vi "Fetch Multi Eval Meas List Segment Modulation Results.vi"(6 "Segment (1)":T2=1, 8 "error in (no error)":errorcluster, 9 "Result Type (Current)":i32(ring) items=["Current"=0, "Average"=1, "Standard Deviation"=3], 10 "Instance (1)":T3=1, 11 "VISA resource name":refnum<visa-resource-name>) -> (0 "error out":errorcluster, 1 "Results":dbl[](array[numeric]) format="%^.3e", 2 "Reliability":T1, 3 "VISA resource name out":refnum<visa-resource-name>, 4 "Expired Statistics":i32, 5 "Out Of Tolerance":i32)   [LabVIEW 2020, in "Rohde&Schwarz CMWXP NR FR1 Measurement.lvlib"]
doc: "Returns modulation single value results for segment <no> in list mode.\n\nAttributes:\nRSCMWXPNRFR1M_ATTR_FETCH_MULTI_EVAL_MEAS_LIST_SEGMENT_MODULATION_CURRENT_RESULTS\nRSCMWXPNRFR1M_ATTR_FETCH_MULTI_EVAL_MEAS_LIST_SEGMENT_MODULATION_AVERAGE_RESULTS\nRSCMWXPNRFR1M_ATTR_FETCH_MULTI_EVAL_MEAS_LIST_SEGMENT_MODULATION_STANDARD_DEVIATION_RESULTS\n\nRemote-control commands:\nFETCh:NRSub:MEAS<i>:MEValuation:LIST:SEGMent<no>:MODulation:CURRent?\nFETCh:NRSub:MEAS<i>:MEValuation:LIST:SEGMent<no>:MODulation:AVERage?\nFETCh:NRSub:MEAS<i>:MEValuation:LIST:SEGMent<no>:MODulation:SDEViation?"
uses:
  <instrlib>/Rohde&Schwarz CMWXP NR FR1 Measurement/Rohde&Schwarz CMWXP NR FR1 Measurement.lvlib
  <instrlib>/Rohde&Schwarz CMWXP NR FR1 Measurement/Private/_Instance.ctl
  <instrlib>/Rohde&Schwarz CMWXP NR FR1 Measurement/Private/_Segment.ctl
  <instrlib>/Rohde&Schwarz CMWXP NR FR1 Measurement/Private/_SegReliability.ctl
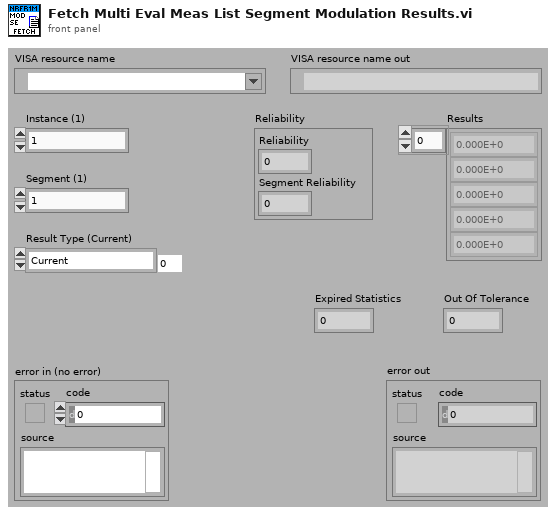
[diagram p1: front panel]
types:
  T1 = typedef "Rohde&Schwarz CMWXP NR FR1 Measurement.lvlib/_SegReliability.ctl" = cluster{"Reliability":i32, "Segment Reliability":i32}
  T2 = typedef "Rohde&Schwarz CMWXP NR FR1 Measurement.lvlib/_Segment.ctl" = i32
  T3 = typedef "Rohde&Schwarz CMWXP NR FR1 Measurement.lvlib/_Instance.ctl" = i32
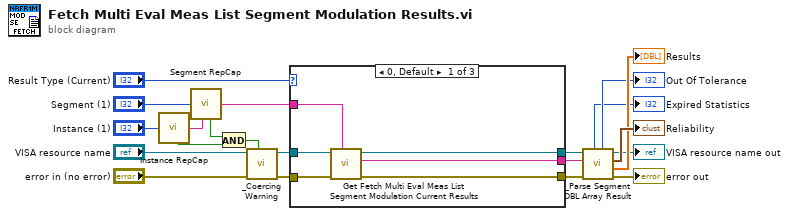
[diagram p0: block diagram]
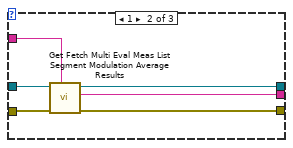
[diagram p2: hidden frame]
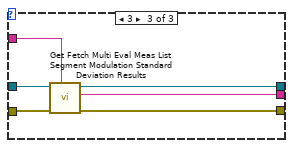
[diagram p3: hidden frame]
diagram:
  n1 = call <instrlib>:"Instance RepCap.vi"("Instance In"="Instance (1)") -> ("In Range?"=w16:bool, "RepCap Identifier Out"=w15:string)  [unwired: 1 in]
  n2 = call <instrlib>:"Segment RepCap.vi"("Segment In"="Segment (1)", "RepCap String In (\"\")"=w15) -> ("In Range?"=w14:bool, "RepCap Identifier Out"=w13:string)
  n3 = And(x=w14, y=w16) -> (x .and. y?=w17:bool)
  n4 = call <instrlib>:"_Coercing Warning.vi"("In Range?"=w17, "error in (no error)"="error in (no error)", "VISA resource name"="VISA resource name") -> ("error out"=w11:errorcluster, "VISA resource name out"=w12:refnum<visa-resource-name>)  [unwired: 7 in]
  n5 = case shown="0, Default" "Result Type (Current)" {
    tunnel: w13 -> [w27 w33 w39]
    tunnel: w12 -> [w26 w32 w38]
    tunnel: w11 -> [w25 w31 w37]
    tunnel: [w24 w30 w36] -> w7
    tunnel: [w23 w29 w35] -> w8
    tunnel: [w22 w28 w34] -> w9
    frame 0, Default {
      n6 = call "Get Fetch Multi Eval Meas List Segment Modulation Current Results"("Repeated Capabilities"=w27, "error in (no error)"=w25, "instrument handle"=w26) -> ("error out"=w22:errorcluster, "Fetch Multi Eval Meas List Segment Modulation Current Results"=w23:string, "instrument handle out"=w24:refnum<visa-resource-name>)  [unwired: 6 in]
    }
    frame 1 {
      n7 = call "Get Fetch Multi Eval Meas List Segment Modulation Average Results"("Repeated Capabilities"=w33, "error in (no error)"=w31, "instrument handle"=w32) -> ("error out"=w28:errorcluster, "Fetch Multi Eval Meas List Segment Modulation Average Results"=w29:string, "instrument handle out"=w30:refnum<visa-resource-name>)  [unwired: 6 in]
    }
    frame 3 {
      n8 = call "Get Fetch Multi Eval Meas List Segment Modulation Standard Deviation Results"("Repeated Capabilities"=w39, "error in (no error)"=w37, "instrument handle"=w38) -> ("error out"=w34:errorcluster, "Fetch Multi Eval Meas List Segment Modulation Standard Deviation Results"=w35:string, "instrument handle out"=w36:refnum<visa-resource-name>)  [unwired: 6 in]
    }
  }
  n9 = call <instrlib>:"_Parse Segment DBL Array Result.vi"("error in (no error)"=w9, "Input String"=w8, "VISA resource name"=w7) -> ("error out"=→"error out":errorcluster, "Results"=→"Results":dbl[], "Reliability Results"=→"Reliability":T1, "VISA resource name out"=→"VISA resource name out":refnum<visa-resource-name>, "Out Of Tolerance"=→"Out Of Tolerance":i32, "Statistic Expired"=→"Expired Statistics":i32)  [unwired: 3 in]
